vi "quantizzatore_unipolare.vi"(8 "Segnale input":waveform(dbl), 9 "B (# Bits)":dbl, 10 "Vfs":dbl) -> (0 "Livelli":dbl[](array[numeric]), 1 "Segnale quantizzato":waveform(dbl), 2 "2^B":dbl, 3 "Q":dbl)   [LabVIEW 2009]
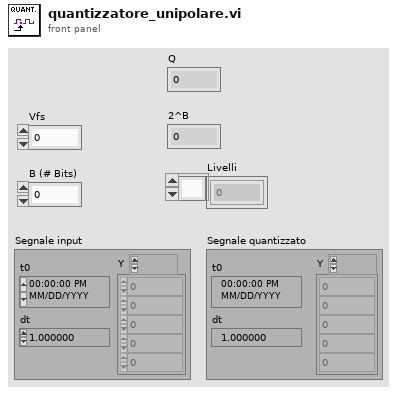
[diagram p1: front panel]
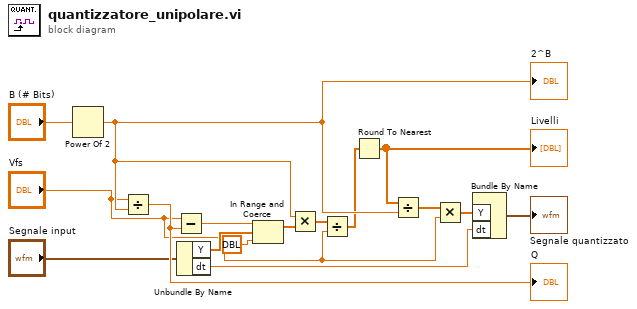
[diagram p0: block diagram]
diagram:
  n1 = Power Of 2(x="B (# Bits)") -> (2^x=w13:dbl)
  "2^B" <- w13
  n2 = Divide(x="Vfs", y=w13) -> (x/y=w16:dbl)
  "Q" <- w16
  n3 = Subtract(x="Vfs", y=w16) -> (x-y=w5:dbl)
  n4 = Unbundle By Name("Segnale input") -> ("Y"=w11:dbl[], "dt"=w9:dbl)
  n5 = In Range and Coerce(upper limit=w5, x=w11, lower limit=dbl ?) -> (coerced(x)=w4:dbl[])  [unwired: 1 out]
  n6 = Multiply(x=w13, y=w4) -> (x*y=w3:dbl[])
  n7 = Divide(x=w3, y="Vfs") -> (x/y=w2:dbl[])
  n8 = Round To Nearest(number=w2) -> (nearest integer value=w7:dbl[])
  "Livelli" <- w7
  n9 = Divide(x=w7, y=w13) -> (x/y=w15:dbl[])
  n10 = Multiply(x=w15, y="Vfs") -> (x*y=w10:dbl[])
  n11 = Bundle By Name("Y"=w10, "dt"=w9) -> (→"Segnale quantizzato":waveform(dbl))  [unwired: 1 in]
